vi "Get Parameter Information.vi"(8 "error in":errorcluster, 11 "variant data":variant) -> (0 "error out":errorcluster, 1 "repeated":bool, 2 "grpc type":T1, 3 "name":string, 4 "message type":string)   [LabVIEW 2021, in "NI Measurement Plug-In SDK.lvlib"]
uses:
  NI Measurement Plug-In SDK.lvlib
  TypeDefs/Google Protobuf Field Kind.ctl
  <vilib>/Utility/Data Type/NI_Data Type.lvlib
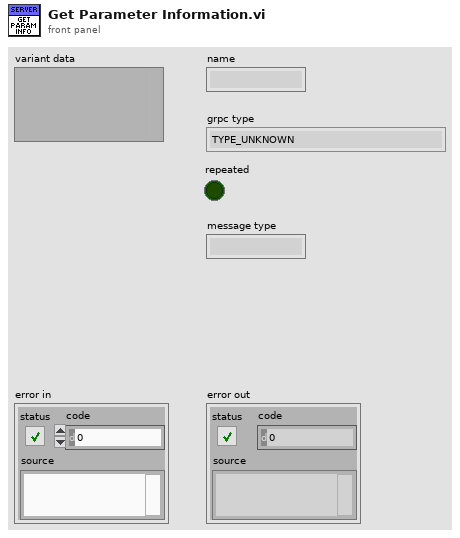
[diagram p1: front panel]
types:
  T1 = typedef "NI Measurement Plug-In SDK.lvlib/Google Protobuf Field Kind.ctl" = enum32{"TYPE_UNKNOWN", "TYPE_DOUBLE", "TYPE_FLOAT", "TYPE_INT64", "TYPE_UINT64", "TYPE_INT32", "TYPE_FIXED64", "TYPE_FIXED32", "TYPE_BOOL", "TYPE_STRING", "TYPE_GROUP", "TYPE_MESSAGE", "TYPE_BYTES", "TYPE_UINT32", "TYPE_ENUM", "TYPE_SFIXED32", "TYPE_SFIXED64", "TYPE_SINT32", "TYPE_SINT64"}
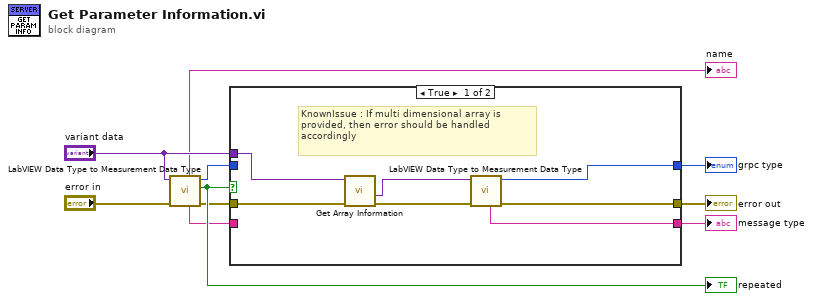
[diagram p0: block diagram]
diagram:
  n1 = call "LabVIEW Data Type to Measurement Data Type.vi"("error in"="error in", "variant"="variant data") -> ("error out"=w2:errorcluster, "array?"=w10:bool, "grpc type"=w1:T1, "message type"=w6:string, "name"=→"name":string)  [unwired: 4 in, 1 out]
  "repeated" <- w10
  n2 = case shown="True" w10 {
    tunnel: w1 -> [_ w19]
    tunnel: w2 -> [w17 w20]
    tunnel: "variant data" -> [w16 _]
    tunnel: [w15 w20] -> w3
    tunnel: w6 -> [_ w18]
    tunnel: [w14 w19] -> w8
    tunnel: [w13 w18] -> w9
    frame True {
      # "KnownIssue : If multi dimensional array is provided, then error should be handled accordingly"
      n3 = call <vilib>:"Get Array Information.vi"("error in (no error)"=w17, "variant"=w16) -> ("error out"=w12:errorcluster, "array element data type"=w11:variant)  [unwired: 6 in, 2 out]
      n4 = call "LabVIEW Data Type to Measurement Data Type.vi"("error in"=w12, "variant"=w11) -> ("error out"=w15:errorcluster, "grpc type"=w14:T1, "message type"=w13:string)  [unwired: 4 in, 3 out]
    }
    frame False {
    }
  }
  "message type" <- w9
  "grpc type" <- w8
  "error out" <- w3
